vi "Loadcell_configuration_REV0_2019_02_25.vi"(8 "error in":errorcluster) -> (0 "error out":errorcluster, 3 "task out":refnum<k21>)   [LabVIEW 2017]
uses:
  <vilib>/DAQmx/create/channels.llb/DAQmx Create Channel (AI-Bridge).vi
  <resource>/objmgr/daqmx.rc
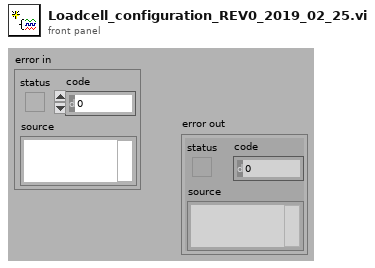
[diagram p1: front panel]
types:
  T1 = cluster{"bridge configuration":i32, "voltage excitation source":i32, "voltage excitation value":dbl, "nominal bridge resistance":dbl}
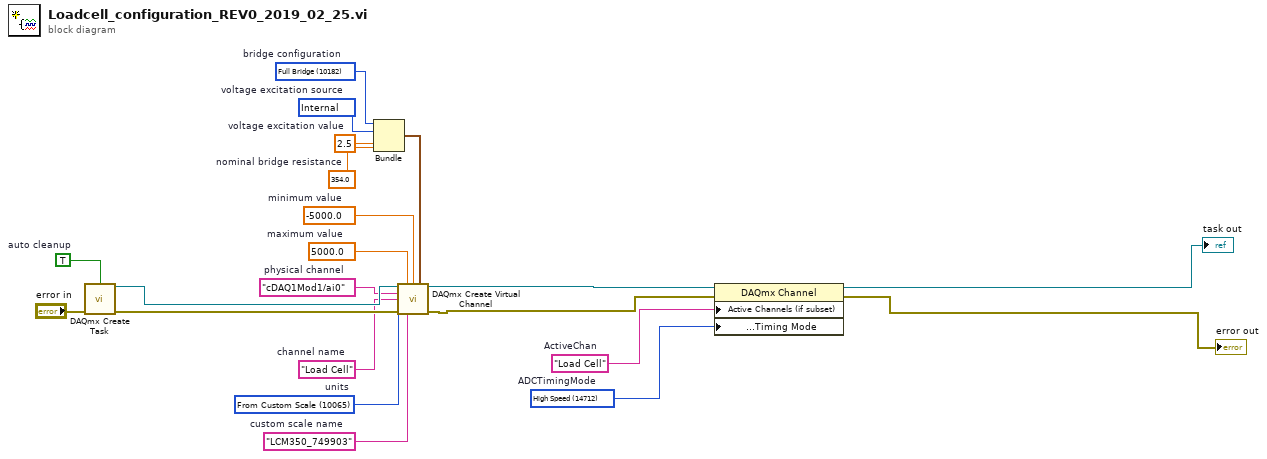
[diagram p0: block diagram]
diagram:
  w4 = 14712 items=["High Resolution"=10195, "High Speed"=14712, "Best 50 Hz Rejection"=14713, "Best 60 Hz Rejection"=14714]  # ADCTimingMode
  w5 = "Load Cell"  # ActiveChan
  w6 = 10065 items=["Volts/Volt"=15896, "mVolts/Volt"=15897, "From Custom Scale"=10065]  # units
  w7 = 354.0  # nominal bridge resistance
  w8 = 2.5  # voltage excitation value
  w9 = 10200 items=["None"=10230, "Internal"=10200, "External"=10167]  # voltage excitation source
  w10 = 10182 items=["Full Bridge"=10182, "Half Bridge"=10187, "Quarter Bridge"=10270]  # bridge configuration
  w12 = "Load Cell"  # channel name
  w14 = "LCM350_749903"  # custom scale name
  w15 = -5000.0  # minimum value
  w16 = 5000.0  # maximum value
  w17 = "cDAQ1Mod1/ai0"  # physical channel
  w19 = TRUE  # auto cleanup
  n1 = call <vilib>:"DAQmx Create Task.vi"("auto cleanup"=w19, "error in"="error in") -> ("task out"=w18:refnum<k21>, "error out"=w20:errorcluster)  [unwired: 12 in]
  n2 = Bundle("bridge configuration"=w10, "voltage excitation source"=w9, "voltage excitation value"=w8, "nominal bridge resistance"=w7) -> (w11:T1)  [unwired: 1 in]
  n3 = call-poly <vilib>:"DAQmx Create Virtual Channel.vi"("task in"=w18, "maximum value"=w16, "minimum value"=w15, "bridge information"=w11, "physical channels"=w17, "name to assign"=w12, "units"=w6, "error in"=w20, "custom scale name"=w14) -> ("task out"=w3:refnum<k21>, "error out"=w13:errorcluster)  [unwired: 5 in]
  n4 = property class="DAQmx Channel"(reference=w3, error in=w13, "Active Channels (if subset)"=w5, "Analog Input:General Properties:Digitizer/ADC:Timing Mode"=w4) -> (reference out=→"task out":refnum<k21>, error out=→"error out":errorcluster)
